vi "cRIO_onboard_laser_read.vi"() -> ()   [LabVIEW 2020]
uses:
  <vilib>/Platform/TimedLoop/XDataNode/timing_clust.ctl
  <vilib>/Platform/TimedLoop/XDataNode/nitl_modes.ctl
  <vilib>/Platform/TimedLoop/XDataNode/wakeup.ctl
  <vilib>/Platform/TimedLoop/XDataNode/loadnilvce.vi
  <vilib>/platform/TimedLoop/XDataNode/XDataNode.xnode
  <vilib>/Platform/TimedLoop/XDataNode/XDNodeRunTimeDep.lvlib
panel:
  out "Readout (V)":dbl[][](array[numeric])
  out "Laser Displacement - cRIO (onboard execution)":dbl[][](graph)
  in  "stop":bool
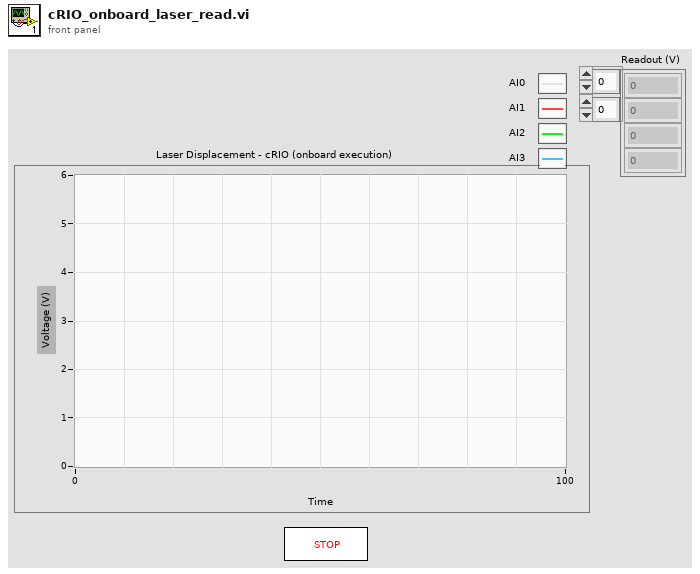
[diagram p1: front panel]
types:
  T1 = typedef "XDNodeRunTimeDep.lvlib/timing_clust.ctl" = cluster{"Expected End [f-1]":u64, "Actual End [f-1]":u64, "Finished Late? [f-1]":bool, "Expected End [i-1]":u64, "Actual End [i-1]":u64, "Finished Late? [i-1]":bool, "Expected Start [i]":u64, "Actual Start [i]":u64, "Expected Start [f]":u64, "Actual Start [f]":u64, "Source Name":string, "Structure Name":string, "Period":i64, "Deadline":i64, "Offset":i64, "Start":i64, "Priority":i32, "Timeout":i32, "Mode":T2, "Wakeup Reason":T3, "Error":errorcluster, "Source Type":string, "Secondary Source Type":string, "Global End Time":u64, "Global Start Time":u64, "Frame Duration":u64, "Iteration Duration":u64, "Assigned CPU":i32, "I/O Scan Engine Mode":u32}
  T2 = typedef "XDNodeRunTimeDep.lvlib/nitl_modes.ctl" = enum32{"No Change", "Process missed periods, maintain original phase", "Discard missed periods, maintain original phase", "Process missed periods, ignore original phase", "Discard missed periods, ignore original phase"}
  T3 = typedef "XDNodeRunTimeDep.lvlib/wakeup.ctl" = enum32{"Normal", "Aborted", "Asynchronous wakeup", "Timing source error", "Timed loop error", "Timeout"}
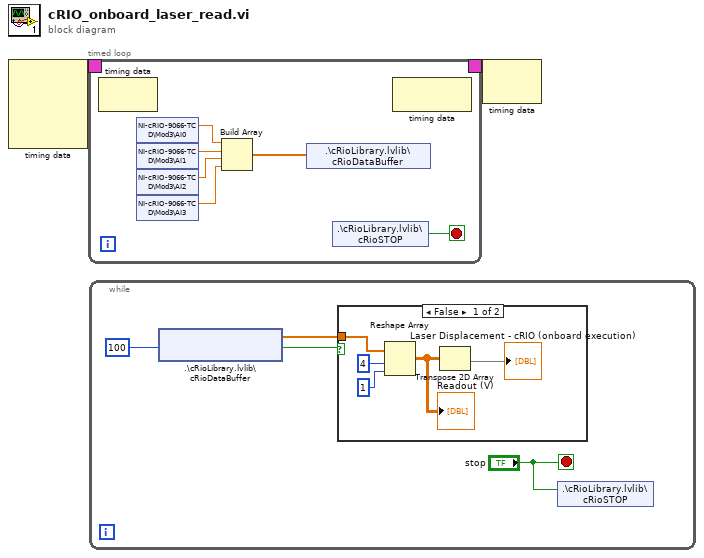
[diagram p0: block diagram]
diagram:
  n1 = node-c288() -> (w2:T1)  [unwired: 4 in]
  n2 = timed-loop {
    timing: w2 -> [_]
    timing-out: [_] -> w1
    stop <- w3 stop-if-true
    n3 = node-c288() -> ()  [unwired: 1 in, 1 out]
    n4 = shared-variable "NI-cRIO-9066-TCD\\Mod3\\AI0"() -> (w8:dbl)  [unwired: 1 in, 1 out]
    n5 = shared-variable "NI-cRIO-9066-TCD\\Mod3\\AI1"() -> (w5:dbl)  [unwired: 1 in, 1 out]
    n6 = shared-variable "NI-cRIO-9066-TCD\\Mod3\\AI2"() -> (w7:dbl)  [unwired: 1 in, 1 out]
    n7 = shared-variable "NI-cRIO-9066-TCD\\Mod3\\AI3"() -> (w6:dbl)  [unwired: 1 in, 1 out]
    n8 = Build Array(w8, w5, w7, w6) -> (w4:dbl[])
    n9 = shared-variable ".\\cRioLibrary.lvlib\\cRioDataBuffer"(w4) -> ()  [unwired: 1 in, 1 out]
    n10 = shared-variable ".\\cRioLibrary.lvlib\\cRioSTOP"() -> (w3:bool)  [unwired: 1 in, 1 out]
    n11 = node-c288() -> ()  [unwired: 1 in, 1 out]
  }
  n12 = while {
    stop <- "stop" stop-if-true
    n13 = shared-variable ".\\cRioLibrary.lvlib\\cRioDataBuffer"(100) -> (w13:dbl[], w11:bool)  [unwired: 1 in, 1 out]
    n14 = case shown="False" w11 {
      tunnel: w13 -> [w17 _]
      frame False {
        n15 = Reshape Array(w17, 4 ("dimension size"), 1 ("dimension size")) -> (w15:dbl[][])
        "Readout (V)" <- w15
        n16 = Transpose 2D Array(2D array=w15) -> (transposed array=→"Laser Displacement - cRIO (onboard execution)":dbl[][])
      }
      frame True {
        # "FIFO empty\nDo nothing"
      }
    }
    n17 = shared-variable ".\\cRioLibrary.lvlib\\cRioSTOP"("stop") -> ()  [unwired: 1 in, 1 out]
  }
  n18 = node-c288(w1) -> ()  [unwired: 1 out]
